vi "Read Center Orientation.vi"(7 "config_in":T2, 8 "error in":errorcluster, 9 "position":i32, 10 "chuck":i32, 11 "Section":string) -> (0 "error out":errorcluster, 2 "Location/Orientation":T1, 5 "config_out":T2)   [LabVIEW 2011]
uses:
  <vilib>/Utility/config.llb/Config Data RefNum.ctl
  Type Definitions/Position_Orientation.ctl
  Vec3d Class/Vec3d Class.lvclass
  <vilib>/Utility/config.llb/Read Key (String).vi
  <vilib>/Utility/config.llb/NI_LVConfig.lvlib
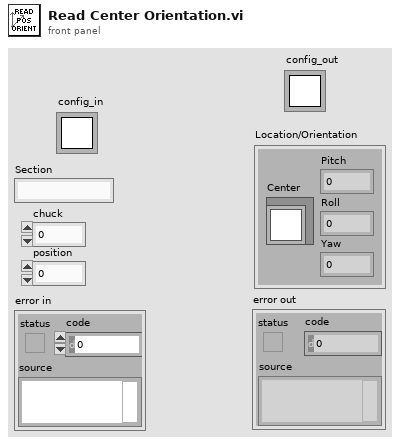
[diagram p1: front panel]
types:
  T1 = typedef "Position_Orientation.ctl" = cluster{"Center":refnum<class "Vec3d Class.lvclass">, "Pitch":dbl, "Roll":dbl, "Yaw":dbl}
  T2 = typedef "NI_LVConfig.lvlib/Config Data RefNum.ctl" = refnum<k1>
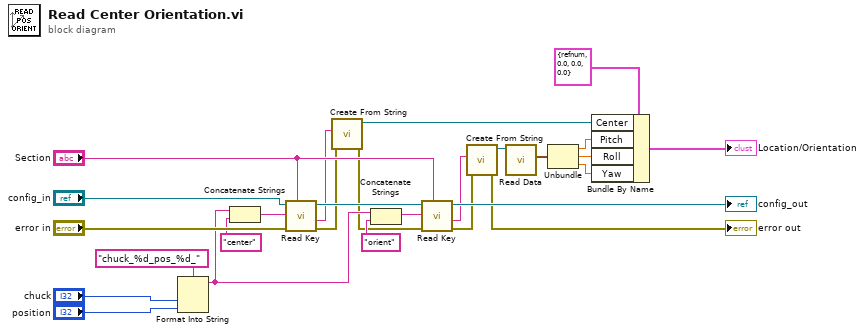
[diagram p0: block diagram]
diagram:
  n1 = Format Into String(format string="chuck_%d_pos_%d_", "chuck", "position") -> (resulting string=w11:string)  [unwired: 2 in, 1 out]
  n2 = Concatenate Strings(w11, "center" ("string")) -> (w13:string)
  n3 = call-poly <vilib>:"Read Key.vi"("section"="Section", "error in (no error)"="error in", "key"=w13, "refnum"="config_in") -> ("error out"=w8:errorcluster, "value"=w10:string, "refnum out"=w25:T2)  [unwired: 4 in, 1 out]
  n4 = call "Create From String.vi"("error in (no error)"=w8, "Input String"=w10) -> ("error out"=w7:errorcluster, "Vec3d Class out"=w9:refnum<class "Vec3d Class.lvclass">)  [unwired: 8 in]
  n5 = Concatenate Strings(w11, "orient" ("string")) -> (w12:string)
  n6 = call-poly <vilib>:"Read Key.vi"("section"="Section", "error in (no error)"=w7, "key"=w12, "refnum"=w25) -> ("error out"=w2:errorcluster, "value"=w3:string, "refnum out"=→"config_out":T2)  [unwired: 4 in, 1 out]
  n7 = call "Create From String.vi"("error in (no error)"=w2, "Input String"=w3) -> ("error out"=→"error out":errorcluster, "Vec3d Class out"=w18:refnum<class "Vec3d Class.lvclass">)  [unwired: 8 in]
  n8 = call-dynamic "Read Data.vi"("Vec3d Class in"=w18) -> ("Data"=w17:cluster{"X":dbl, "Y":dbl, "Z":dbl})  [unwired: 8 in, 2 out]
  n9 = Unbundle(w17) -> ("X"=w6:dbl, "Y"=w5:dbl, "Z"=w4:dbl)
  n10 = Bundle By Name(cluster=T1 {"Center"=refnum, "Pitch"=0.0, "Roll"=0.0, "Yaw"=0.0} ("Location/Orientation"), "Center"=w9, "Pitch"=w6, "Roll"=w5, "Yaw"=w4) -> (→"Location/Orientation":T1)
